vi "GasflaschenHeader_Kopfzeile_einfuegen.vi"(11 "Array (Eingang)":T1[][](array[typedef])) -> (3 "Array (Ausgang)":T1[][](array[typedef]))   [LabVIEW 2020, in "System Einstellungen V2.lvlib"]
uses:
  System Einstellungen V2.lvlib
  Traegergas.ctl
  Sprachverwaltung/FGV Aktion Tabelle zerlegen.ctl
  Sprachverwaltung/Sprachverwaltung.lvlib
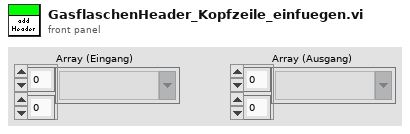
[diagram p1: front panel]
types:
  T1 = typedef "System Einstellungen V2.lvlib/Traegergas.ctl" = string
  T2 = typedef "Sprachverwaltung.lvlib/FGV Aktion Tabelle zerlegen.ctl" = enum16{"laden", "vereinzeln", "speichern"}
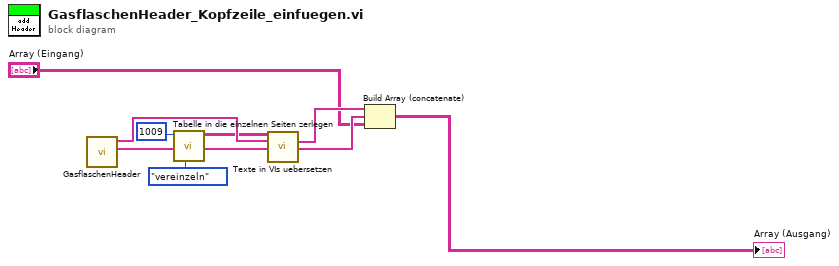
[diagram p0: block diagram]
diagram:
  n1 = call "GasflaschenHeader.vi"() -> ("Trennlinie"=w8:string[], "Header"=w4:string[])  [unwired: 10 in]
  n2 = call "Tabelle in die einzelnen Seiten zerlegen.vi"("Aktion"=FGV_Aktion_Tabelle_zerlegen."vereinzeln", "Index (Seite)"=1009) -> ("Sprachliste"=w3:string[][])  [unwired: 7 in, 2 out]
  n3 = call "Texte in VIs uebersetzen.vi"("Sprachliste"=w3, "String-Array zum Übersetzen"=w4) -> ("String-Array zum Übersetzen"=w7:string[])  [unwired: 9 in, 4 out]
  n4 = Build Array (concatenate)(w7, w8, "Array (Eingang)") -> (→"Array (Ausgang)":T1[][])
